vi "Log CSV PassFail Data.vi"(7 "Source CSV Path":path, 8 "Error In":errorcluster, 10 "Options":T1, 11 "Log Data":string[][](array[string])) -> (0 "Error Out":errorcluster)   [LabVIEW 2011]
uses:
  Controls/Options.ctl
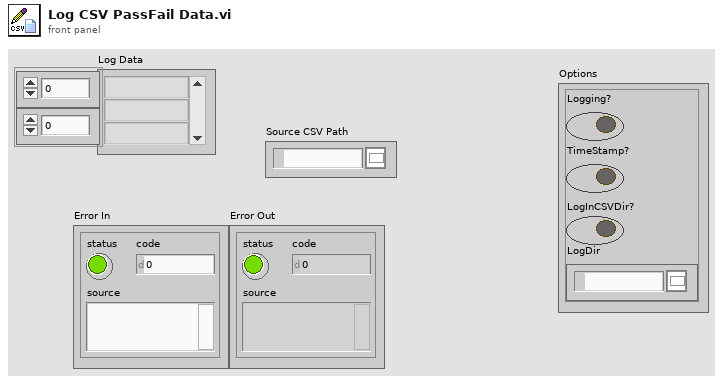
[diagram p1: front panel]
types:
  T1 = typedef "Options.ctl" = cluster{"Logging?":bool, "TimeStamp?":bool, "LogInCSVDir?":bool, "LogDir":path}
  T2 = enum16{"open", "replace", "create", "open or create", "replace or create", "replace or create with confirmation"}
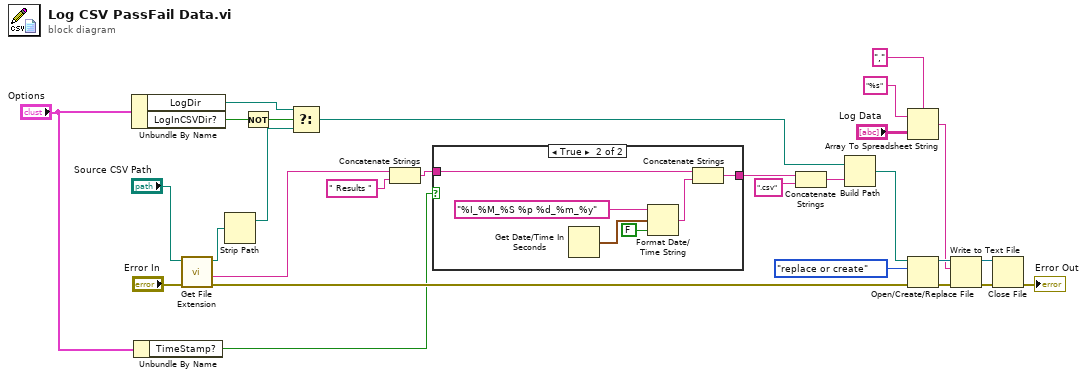
[diagram p0: block diagram]
diagram:
  n1 = Unbundle By Name("Options") -> ("LogDir"=w3:path, "LogInCSVDir?"=w13:bool)
  n2 = Unbundle By Name("Options") -> ("TimeStamp?"=w5:bool)
  n3 = call <vilib>:"Get File Extension.vi"("error in (no error)"="Error In", "file"="Source CSV Path") -> ("error out"=w14:errorcluster, "filename without extension"=w16:string, "dup file"=w4:path)  [unwired: 6 in, 1 out]
  n4 = Strip Path(path=w4) -> (stripped path=w2:path)  [unwired: 1 out]
  n5 = Not(x=w13) -> (.not. x?=w12:bool)
  n6 = Select(t=w3, s=w12, f=w2) -> (s? t:f=w1:path)
  n7 = Concatenate Strings(w16, " Results " ("string")) -> (w8:string)
  n8 = case shown="True" w5 {
    tunnel: w8 -> [w29 w35]
    tunnel: [w29 w34] -> w7
    frame False {
    }
    frame True {
      n9 = Get Date/Time In Seconds() -> (seconds since 1Jan1904=w31:timestamp)
      n10 = Format Date/Time String(time format string (%c)="%I_%M_%S %p %d_%m_%y", seconds (now)=w31, UTC format=FALSE) -> (date/time string=w30:string)
      n11 = Concatenate Strings(w35, w30) -> (w34:string)
    }
  }
  n12 = Concatenate Strings(w7, ".csv" ("string")) -> (w9:string)
  n13 = Build Path(base path=w1, name or relative path=w9) -> (appended path=w15:path)
  n14 = Array To Spreadsheet String(delimiter (Tab)=",", array="Log Data", 3:"%s" ("format string")) -> (spreadsheet string=w21:string)
  n15 = Open/Create/Replace File(file path (use dialog)=w15, error in=w14, operation (0:open)=T2."replace or create") -> (refnum out=w25:refnum<file>, error out=w28:errorcluster)  [unwired: 3 in, 1 out]
  n16 = Write to Text File(file (use dialog)=w25, text=w21, error in=w28) -> (refnum out=w26:refnum<file>, error out=w27:errorcluster)  [unwired: 1 in, 1 out]
  n17 = Close File(refnum=w26, error in=w27) -> (error out=→"Error Out":errorcluster)  [unwired: 1 out]
